vi "GetNowTime.vi"() -> (0 "NowTime":string)   [LabVIEW 2012]
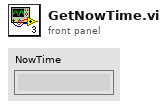
[diagram p1: front panel]
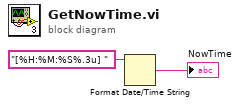
[diagram p0: block diagram]
diagram:
  n1 = Format Date/Time String(time format string (%c)="[%H:%M:%S%.3u] " ("时间格式字符串(%c)")) -> (date/time string=→"NowTime":string)  [unwired: 2 in]
